vi "Test_peregrine.vi"() -> ()   [LabVIEW 2019]
panel:
  in  "Acceleration\n(moveS)":u16
  in  "Speed\n(moveS)":i16
  in  "Target\n(moveS)":i32
  out "Speed response\n(moveS)":i16
  out "Position response\n(moveS)":i32
  out "Flags\nmoveS":T1
  out "Value response\n(write)":i32
  out "Key response\n(write)":u32
  in  "Value\n(write)":i32
  in  "Key\n(write)":u32
  out "Value response\n(read)":i32
  out "Key response\n(read)":u32
  in  "Value\n(read)":i32
  in  "Key\n(read)":u32
  in  "Speed\n(move)":i16
  in  "Acceleration\n(move)":u16
  in  "Target\n(move(":i32
  out "Flags\n(query)":T1
  out "Position\n(query)":i32
  out "Speed\n(query)":i16
  in  "Address":u8
  in  "COM Port for serial\nconnection. Check device\nmanager.":string
  # "Peregrine test program for move+query+write+read"
  # "Move with Status\nrespones"
  # "General inputs"
  # "Query responses"
  # "Read responses"
  # "Move with status\ninputs"
  # "Move inputs"
  # "Write responses"
  # "Read inputs"
  # "Write inputs"
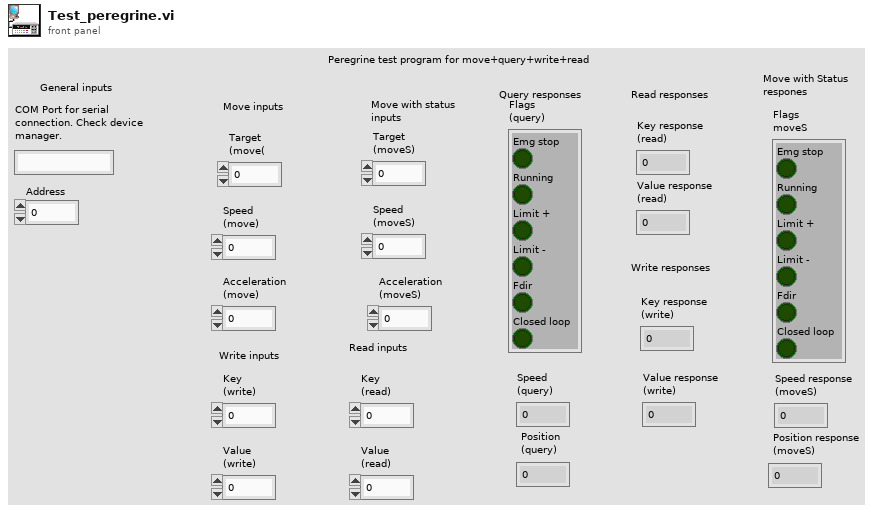
[diagram p1: front panel]
types:
  T1 = cluster{"Emg stop":bool, "Running":bool, "Limit +":bool, "Limit -":bool, "Fdir":bool, "Closed loop":bool}
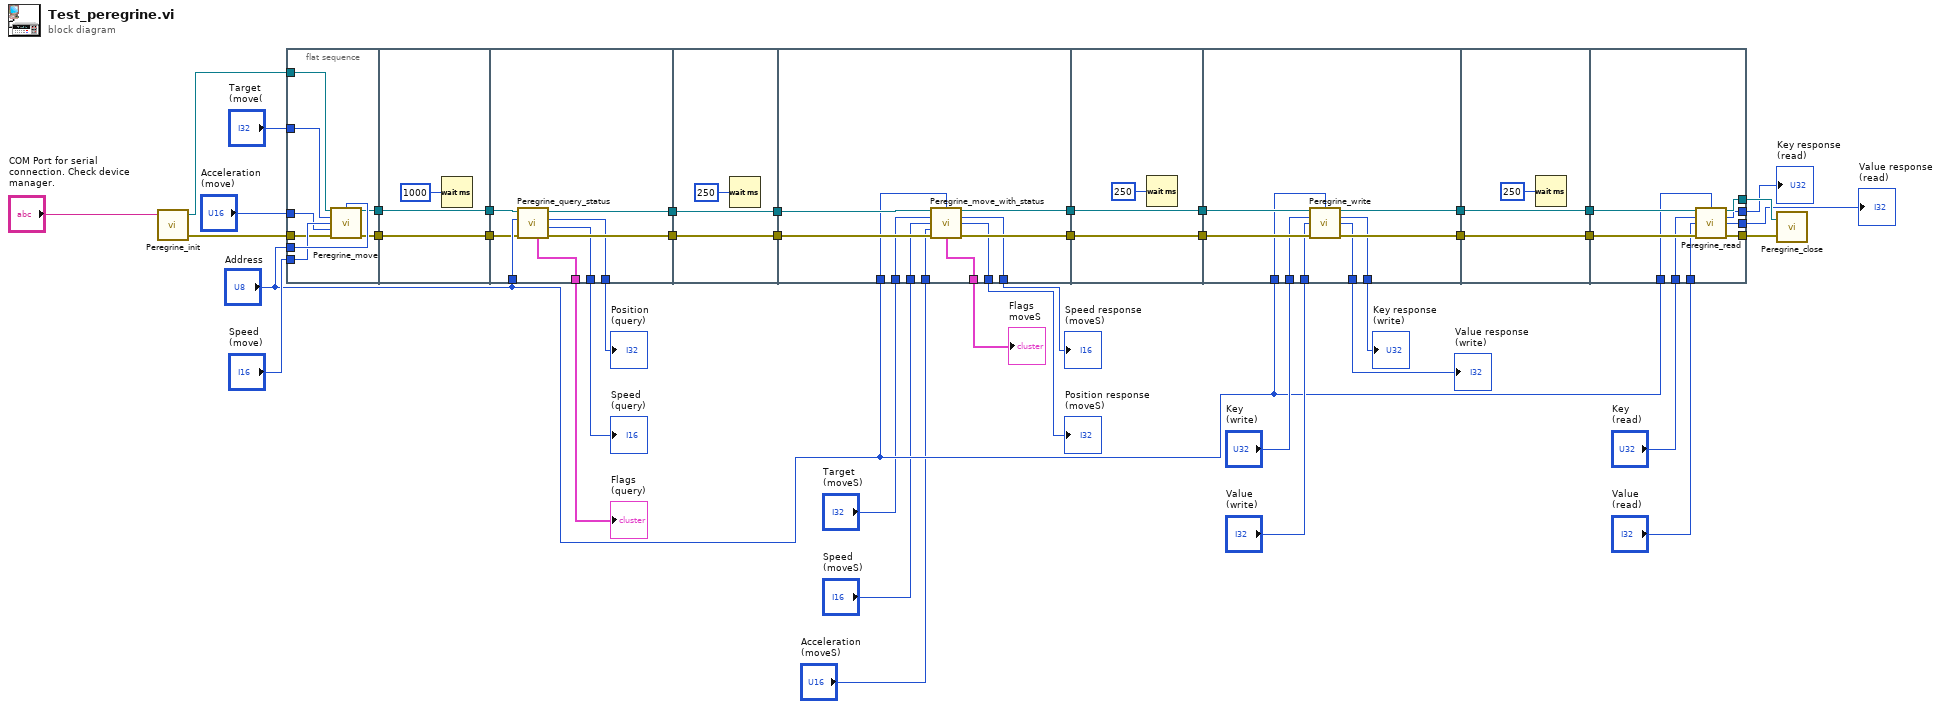
[diagram p0: block diagram]
diagram:
  n1 = call "Peregrine_init.vi"("COM Port for serial\nconnection. Check device\nmanager."="COM Port for serial\nconnection. Check device\nmanager.") -> ("error out"=w37:errorcluster, "Handle out"=w41:refnum<visa-resource-name>)  [unwired: 3 in]
  n2 = flat-sequence {
    tunnel: w41 -> [w50]
    tunnel: "Address" -> [w49]
    tunnel: "Target\n(move(" -> [w48]
    tunnel: "Speed\n(move)" -> [w47]
    tunnel: "Acceleration\n(move)" -> [w46]
    tunnel: w37 -> [w45]
    tunnel: [w44] -> w34
    tunnel: [w43] -> w33
    tunnel: w34 -> [w51]
    tunnel: w33 -> [w52]
    tunnel: [w52] -> w32
    tunnel: [w51] -> w31
    tunnel: "Address" -> [w61]
    tunnel: w32 -> [w57]
    tunnel: w31 -> [w58]
    tunnel: [w60] -> w30
    tunnel: [w59] -> w29
    tunnel: [w56] -> w20
    tunnel: [w55] -> w18
    tunnel: [w54] -> w19
    tunnel: w30 -> [w64]
    tunnel: w29 -> [w63]
    tunnel: [w64] -> w11
    tunnel: [w63] -> w9
    tunnel: w11 -> [w74]
    tunnel: [w73] -> w10
    tunnel: w9 -> [w75]
    tunnel: [w72] -> w8
    tunnel: [w71] -> w7
    tunnel: "Address" -> [w70]
    tunnel: [w69] -> w5
    tunnel: [w68] -> w4
    tunnel: "Target\n(moveS)" -> [w67]
    tunnel: "Speed\n(moveS)" -> [w66]
    tunnel: "Acceleration\n(moveS)" -> [w65]
    tunnel: w10 -> [w78]
    tunnel: [w78] -> w13
    tunnel: w8 -> [w77]
    tunnel: [w77] -> w12
    tunnel: w13 -> [w85]
    tunnel: [w84] -> w24
    tunnel: w12 -> [w87]
    tunnel: [w86] -> w22
    tunnel: "Address" -> [w83]
    tunnel: "Key\n(write)" -> [w82]
    tunnel: "Value\n(write)" -> [w81]
    tunnel: [w80] -> w15
    tunnel: [w79] -> w14
    tunnel: w24 -> [w90]
    tunnel: [w90] -> w23
    tunnel: w22 -> [w89]
    tunnel: [w89] -> w21
    tunnel: [w97] -> w35
    tunnel: [w96] -> w36
    tunnel: w23 -> [w98]
    tunnel: w21 -> [w99]
    tunnel: "Address" -> [w95]
    tunnel: "Key\n(read)" -> [w94]
    tunnel: "Value\n(read)" -> [w93]
    tunnel: [w92] -> w26
    tunnel: [w91] -> w25
    frame #0 {
      n3 = call "Peregrine_move.vi"("Handle in"=w50, "Address"=w49, "Target"=w48, "Speed"=w47, "Acceleration"=w46, "error"=w45) -> ("Handle out"=w43:refnum<visa-resource-name>, "error out"=w44:errorcluster)  [unwired: 8 in]
    }
    frame #1 {
      n4 = Wait (ms)(milliseconds to wait=u32 1000) -> ()  [unwired: 1 out]
    }
    frame #2 {
      n5 = call "Peregrine_query_status.vi"("error"=w58, "Address"=w61, "Handle in"=w57) -> ("error out"=w60:errorcluster, "Speed"=w54:i16, "Position"=w55:i32, "Handle out"=w59:refnum<visa-resource-name>, "Flags"=w56:T1)  [unwired: 4 in]
    }
    frame #3 {
      n6 = Wait (ms)(milliseconds to wait=u32 250) -> ()  [unwired: 1 out]
    }
    frame #4 {
      n7 = call "Peregrine_move_with_status.vi"("Handle in"=w75, "Address"=w70, "Target"=w67, "Speed"=w66, "Acceleration"=w65, "error"=w74) -> ("Handle out"=w72:refnum<visa-resource-name>, "Speed\nresponse"=w68:i16, "Position\nresponse"=w69:i32, "Flags\nmoveS"=w71:T1, "error out"=w73:errorcluster)  [unwired: 5 in]
    }
    frame #5 {
      n8 = Wait (ms)(milliseconds to wait=u32 250) -> ()  [unwired: 1 out]
    }
    frame #6 {
      n9 = call "Peregrine_write.vi"("Handle in"=w87, "Address"=w83, "Key"=w82, "Value"=w81, "error"=w85) -> ("Handle out"=w86:refnum<visa-resource-name>, "Key response"=w80:u32, "Value response"=w79:i32, "error out"=w84:errorcluster)  [unwired: 7 in]
    }
    frame #7 {
      n10 = Wait (ms)(milliseconds to wait=u32 250) -> ()  [unwired: 1 out]
    }
    frame #8 {
      n11 = call "Peregrine_read.vi"("Handle in"=w99, "Address"=w95, "Key"=w94, "Value"=w93, "error"=w98) -> ("Handle out"=w97:refnum<visa-resource-name>, "Key response"=w92:u32, "Value response"=w91:i32, "error out"=w96:errorcluster)  [unwired: 7 in]
    }
  }
  n12 = call "Peregrine_close.vi"("error in (no error)"=w36, "Handle in"=w35) -> ()  [unwired: 1 in, 1 out]
  "Speed\n(query)" <- w19
  "Position\n(query)" <- w18
  "Flags\n(query)" <- w20
  "Key response\n(read)" <- w26
  "Value response\n(read)" <- w25
  "Key response\n(write)" <- w15
  "Value response\n(write)" <- w14
  "Flags\nmoveS" <- w7
  "Position response\n(moveS)" <- w5
  "Speed response\n(moveS)" <- w4
